vi "ExEMCircBufROInframebigbuf.vi"() -> ()   [LabVIEW 2010]
uses:
  CamHandle.vi
panel:
  in  "Number of Images":u32=25
  in  "Start collection":bool
  out "ready to \nstart":bool
  in  "av gain":dbl format="%.2f"
  in  "Invert Logic output":bool
  in  "Logic Output":i32
  in  "Fan":i32=1
  in  "ADC Gain":u32
  out "ADC Speed (Khz)":u32
  in  "Fast ADC":bool
  in  "X Start":u32=1 min=1 step=1
  in  "Y Bin":u32=1 min=1 step=1
  in  "X End":u32=512 min=1 max=512 step=1
  in  "X Bin":u32=1 min=1 step=1
  in  "Y Start":u32=1 min=1 step=1
  in  "Y End":u32=512 min=1 max=512 step=1
  in  "Temperature":dbl=-55.0 format="%.2f"
  in  "Exposure":dbl min=0.0 step=0.001 format="%.3f"
  out "error out":errorcluster
  in  "error in (no error)":errorcluster
  # "ExEMCircBufROInframebigbuf:\nThis example allows a single ROI\nto be programmed up. It then runs\nin sync (nframe)  mode. It  displays \nthe ROI data after all the data comes\nin.\nNote: this example requires the \ncamera support circular buffers.\nThis example also shows how to \nsetup the cascade to run in over-\nlapped mode and how to set the\non-chip multiplication gain and how\nto set the readout port."
  # "Warning: you must open and run once the VI ExOpenGlobalCam.vi.\nYou only need to run it once then you can run this Example VI as many\ntimes as you want."
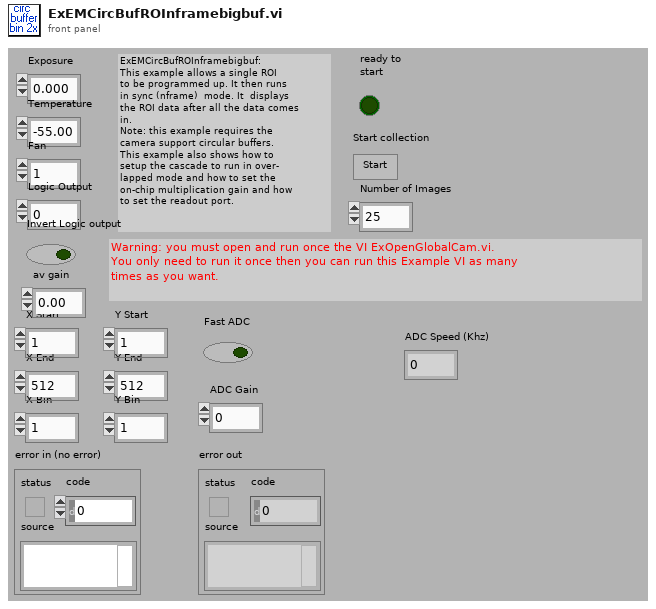
[diagram p1: front panel]
types:
  T1 = cluster{"X Start":u32, "X End":u32, "X Bin":u32, "Y Start":u32, "Y End":u32, "Y Bin":u32}
  T2 = cluster{"acquire focus mode":u32, "Exposure":dbl, "Number of Images":u32, "Software accumulation":u32}
  T3 = cluster{"Camera Handle":u32, "Pulser Handle":u32, "File Handle":u32, "Display Handle":u32, "Image Handle":u32}
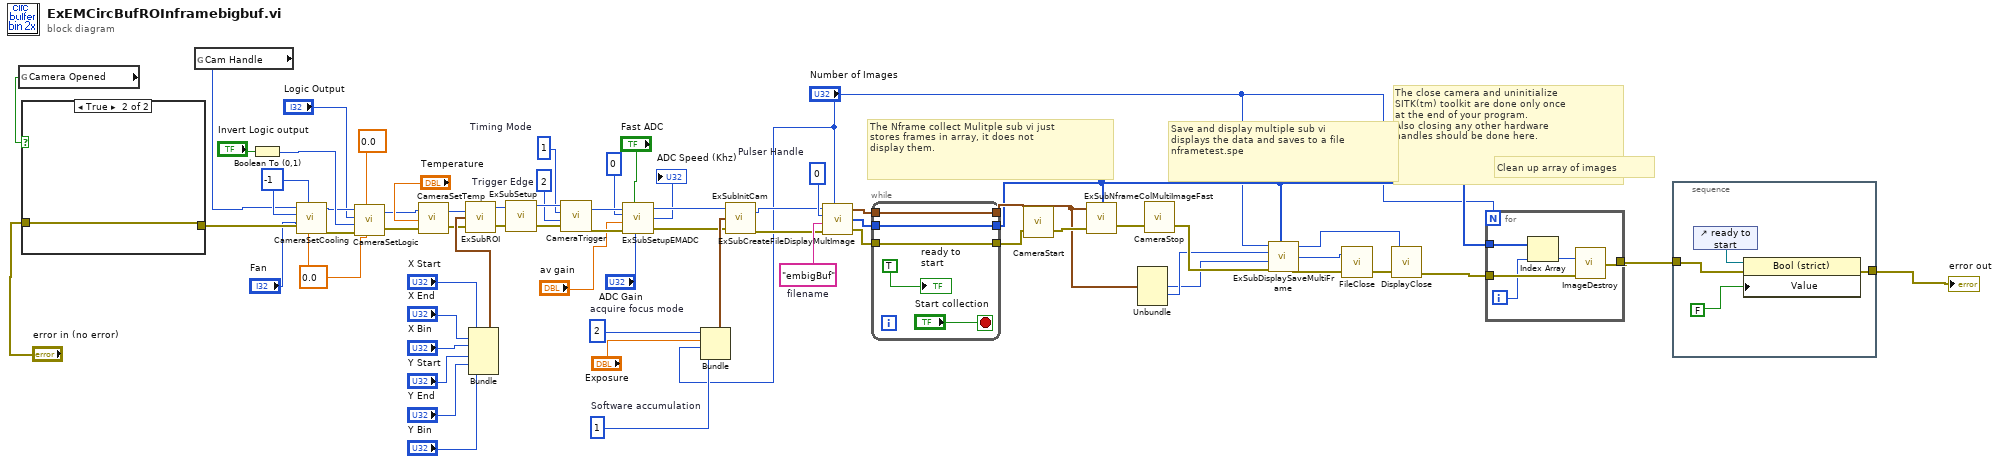
[diagram p0: block diagram]
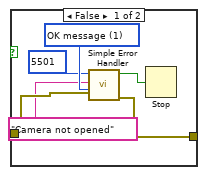
[diagram p2: hidden frame]
diagram:
  w22 = u32 0  # Pulser Handle
  w23 = "embigBuf"  # filename
  w28 = 0.0
  w29 = -1
  w61 = u32 1  # Timing Mode
  w62 = u32 2  # Trigger Edge
  w64 = u32 2  # acquire focus mode
  w63 = u32 1  # Software accumulation
  # "Clean up array of images"
  # "Save and display multiple sub vi\ndisplays the data and saves to a file\nnframetest.spe"
  # "The Nframe collect Mulitple sub vi just \nstores frames in array, it does not \ndisplay them."
  # "The close camera and uninitialize\nSITK(tm) toolkit are done only once\nat the end of your program.\nAlso closing any other hardware \nhandles should be done here."
  n1 = global read "CamHandle.vi" "Camera Opened"() -> (w38:bool)
  n2 = case shown="True" w38 {
    tunnel: "error in (no error)" -> [w72 w74]
    tunnel: [w71 w74] -> w36
    frame False {
      w73 = u16 1 items=["no dialog", "OK message", "continue or stop message"] ("type of dialog (OK msg:1)")
      n3 = call <vilib>:"Simple Error Handler.vi"("error code (no error:0)"=5501, "error source (\" \")"="Camera not opened", "type of dialog (OK msg:1)"=w73, "error in (no error)"=w72) -> ("error?"=w69:bool, "error out"=w71:errorcluster)  [unwired: 1 in, 3 out]
      n4 = Stop(stop? (T)=w69) -> ()
    }
    frame True {
    }
  }
  n5 = global read "CamHandle.vi" "Cam Handle"() -> (w24:u32)
  n6 = Boolean To (0,1)(Boolean="Invert Logic output") -> (0, 1=w32:i16)
  n7 = call <userlib>:"CameraSetCooling.vi"("Reserved"=w28, "Cooling Mode"=w29, "error in (no error)"=w36, "Fan"="Fan", "Cooling"=w29, "Camera Handle"=w24) -> ("error out"=w35:errorcluster, "Camera Handle"=w31:u32)
  n8 = call <userlib>:"CameraSetLogic.vi"("Reserved 2"=w28, "Reserved"=0.0, "error in (no error)"=w35, "Invert Logic"=w32, "Logic Output"="Logic Output", "Camera Handle"=w31) -> ("error out"=w34:errorcluster, "Camera Handle"=w27:u32)
  n9 = call <userlib>:"CameraSetTemp.vi"("error in (no error)"=w34, "Temperature"="Temperature", "Camera Handle"=w27) -> ("error out"=w52:errorcluster, "Camera Handle"=w51:u32)
  n10 = Bundle("X Start"="X Start", "X End"="X End", "X Bin"="X Bin", "Y Start"="Y Start", "Y End"="Y End", "Y Bin"="Y Bin") -> (w54:T1)  [unwired: 1 in]
  n11 = call "ExSubROI.vi"("error in (no error)"=w52, "ROI"=w54, "Camera Handle"=w51) -> ("error out"=w49:errorcluster, "Camera Handle"=w53:u32)
  n12 = call "ExSubSetup.vi"("error in (no error)"=w49, "Camera Handle"=w53) -> ("error out"=w48:errorcluster, "Camera Handle"=w65:u32)
  n13 = call <userlib>:"CameraTrigger.vi"("error in"=w48, "Trigger Edge"=w62, "Timing Mode"=w61, "Camera Handle"=w65) -> ("error out"=w46:errorcluster, "Camera Handle"=w47:u32)
  n14 = call "ExSubSetupEMADC.vi"("Camera Handle"=w47, "Fast ADC"="Fast ADC", "ReadOut Port"=0, "Avalanche Gain\nOnly valid for \nport 0"="av gain", "ADC Gain"="ADC Gain", "error in (no error)"=w46) -> ("Camera Handle"=w44:u32, "ADC Speed (Khz)"=→"ADC Speed (Khz)":u32, "error out"=w45:errorcluster)
  n15 = Bundle("acquire focus mode"=w64, "Exposure"="Exposure", "Number of Images"="Number of Images", "Software accumulation"=w63) -> (w66:T2)  [unwired: 1 in]
  n16 = call "ExSubInitCam.vi"("error in (no error)"=w45, "Camera Information"=w66, "Camera Handle"=w44) -> ("error out"=w4:errorcluster, "Camera Handle"=w5:u32)
  n17 = call "ExSubCreateFileDisplayMultImage.vi"("Camera Handle"=w5, "Pulser Handle"=w22, "File and Display Name"=w23, "error in (no error)"=w4, "Number of Images"="Number of Images") -> ("Handles Out"=w11:T3, "Array"=w7:u32[], "error out"=w9:errorcluster)
  n18 = while {
    tunnel: w11 -> [w79]
    tunnel: [w79] -> w10
    tunnel: w9 -> [w78]
    tunnel: [w78] -> w8
    tunnel: w7 -> [w77]
    tunnel: [w77] -> w6
    stop <- "Start collection" stop-if-true
    "ready to \nstart" <- TRUE
  }
  n19 = call <userlib>:"CameraStart.vi"("error in"=w8) -> ("error out"=w21:errorcluster)  [unwired: 1 in, 1 out]
  n20 = call "ExSubNframeColMultiImageFast.vi"("image handles"=w6, "error in (no error)"=w21, "Handle Cluster"=w10) -> ("error out"=w20:errorcluster)  [unwired: 1 in, 1 out]
  n21 = Unbundle(w10) -> ("File Handle"=w17:u32, "Display Handle"=w18:u32)  [unwired: 3 out]
  n22 = call <userlib>:"CameraStop.vi"("error in"=w20) -> ("error out"=w19:errorcluster)  [unwired: 1 in, 1 out]
  n23 = call "ExSubDisplaySaveMultiFrame.vi"("Number of Images"="Number of Images", "Display Handle"=w18, "file handle"=w17, "error in (no error)"=w19, "Data handles"=w6) -> ("Display Handle"=w12:u32, "file Handle"=w13:u32, "error out"=w14:errorcluster)
  n24 = call <userlib>:"FileClose.vi"("error in"=w14, "File Handle"=w13) -> ("error out"=w16:errorcluster)
  n25 = call <userlib>:"DisplayClose.vi"("error in"=w16, "Display Handle"=w12) -> ("error out"=w15:errorcluster)
  n26 = for {
    N: "Number of Images" -> [_]
    tunnel: w15 -> [w84]
    tunnel: [w83] -> w3
    tunnel: w6 -> [w81]
    i -> [w82]
    n27 = Index Array(array=w81, index=w82) -> (element=w80:u32)
    n28 = call <userlib>:"ImageDestroy.vi"("error in"=w84, "Data handle"=w80) -> ("error out"=w83:errorcluster)
  }
  n29 = stacked-sequence {
    tunnel: w3 -> [w87]
    tunnel: [w85] -> w2
    frame #0 {
      n30 = control-ref of="ready to \nstart"() -> (w88:refnum<vi>)
      n31 = property class="Bool (strict)"(reference=w88, error in=w87, "Value"=FALSE) -> (error out=w85:errorcluster)  [unwired: 1 out]
    }
  }
  "error out" <- w2
